vi "Test LEN.vi"(8 "error in (no error)":errorcluster) -> (0 "error out":errorcluster)   [LabVIEW 2020]
uses:
  Source/Protobuf RAW/string/string.lvclass
  Source/Protobuf RAW/bytes/bytes.lvclass
  Source/Protobuf RAW/string/string.lvclass/string.ctl
  Source/Protobuf RAW/bytes/bytes.lvclass/bytes.ctl
  Source/Protobuf RAW/bytes/Write Value.vi
  Source/Protobuf RAW/string/Write Value.vi
  <vilib>/addons/_JKI Toolkits/Caraya/classes/Assert/Assert Equal Value_Variant.vi
  <vilib>/addons/_JKI Toolkits/Caraya/classes/Test/Test.lvclass
  Source/Protobuf RAW.lvlib
  <vilib>/addons/_JKI Toolkits/Caraya/classes/Assert/Assert.lvclass
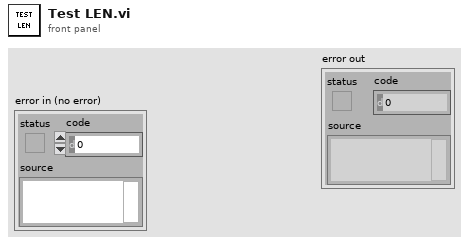
[diagram p1: front panel]
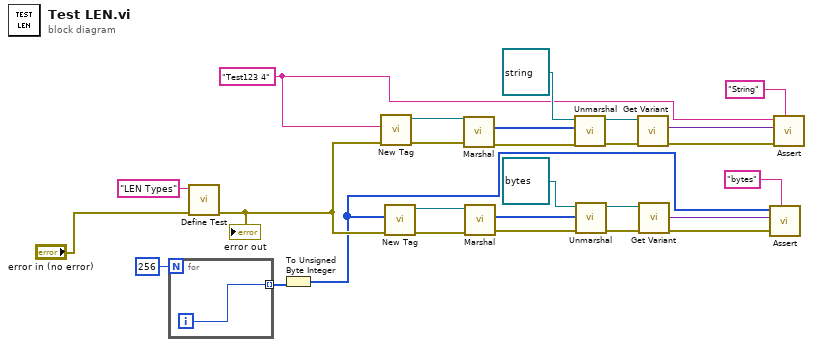
[diagram p0: block diagram]
diagram:
  w2 = "Test123 4" ("Value")
  n1 = for {
    N: 256 -> [_]
    tunnel: [w28] -> w15 mode=indexing
    i -> [w28]
  }
  n2 = call <vilib>:"Define Test.vi"("error in (no error)"="error in (no error)", "Label (VI Title)"="LEN Types") -> ("error out"=w8:errorcluster)  [unwired: 9 in]
  "error out" <- w8
  n3 = To Unsigned Byte Integer(number=w15) -> (unsigned 8bit integer=w6:u8[])
  n4 = call-poly "New Tag.vi"("error in (no error)"=w8, "Value"=w2) -> ("error out"=w24:errorcluster, "string out"=w25:refnum<class "string.lvclass">)  [unwired: 8 in]
  n5 = call-poly "New Tag.vi"("error in (no error)"=w8, "Value"=w6) -> ("error out"=w9:errorcluster, "fixed32 out"=w14:refnum<class "bytes.lvclass">)  [unwired: 8 in]
  n6 = call-dynamic "Marshal.vi"("error in (no error)"=w24, "int32 in"=w25) -> ("error out"=w23:errorcluster, "Buffer"=w22:u8[])  [unwired: 7 in, 1 out]
  n7 = call-dynamic "Marshal.vi"("error in (no error)"=w9, "int32 in"=w14) -> ("error out"=w12:errorcluster, "Buffer"=w11:u8[])  [unwired: 7 in, 1 out]
  n8 = call-dynamic "Unmarshal.vi"("error in (no error)"=w23, "Buffer"=w22, "int32 in"=refnum<class "string.lvclass"> refnum) -> ("error out"=w20:errorcluster, "int32 out"=w19:refnum<class "string.lvclass">)  [unwired: 6 in, 1 out]
  n9 = call-dynamic "Unmarshal.vi"("error in (no error)"=w12, "Buffer"=w11, "int32 in"=refnum<class "bytes.lvclass"> refnum) -> ("error out"=w4:errorcluster, "int32 out"=w13:refnum<class "bytes.lvclass">)  [unwired: 6 in, 1 out]
  n10 = call-dynamic "Get Variant.vi"("error in (no error)"=w20, "int32 in"=w19) -> ("error out"=w18:errorcluster, "Variant"=w3:variant)  [unwired: 7 in, 1 out]
  n11 = call-dynamic "Get Variant.vi"("error in (no error)"=w4, "int32 in"=w13) -> ("error out"=w5:errorcluster, "Variant"=w7:variant)  [unwired: 7 in, 1 out]
  n12 = call-poly <vilib>:"Assert.vi"("Label"="bytes", "error in (no error)"=w5, "Y"=w7, "X"=w6) -> ()  [unwired: 7 in, 1 out]
  n13 = call-poly <vilib>:"Assert.vi"("Label"="String", "error in (no error)"=w18, "Y"=w3, "X"=w2) -> ()  [unwired: 7 in, 1 out]
